vi "Deletar entre Cursores.vi"(8 "error in":errorcluster, 10 "Cluster 3":T1, 11 "WaveformGraph in":refnum<vi>) -> (0 "error out":errorcluster, 2 "output cluster":T1)   [LabVIEW 2020]
uses:
  TypeDef's/Dados consumidor.ctl
  <vilib>/Waveform/WDTOps.llb/WDT Waveform Duration DBL.vi
  <vilib>/Waveform/WDTOps.llb/WDT Get Waveform Subset DBL.vi
  <vilib>/Waveform/WDTOps.llb/WDT Append Waveforms DBL.vi
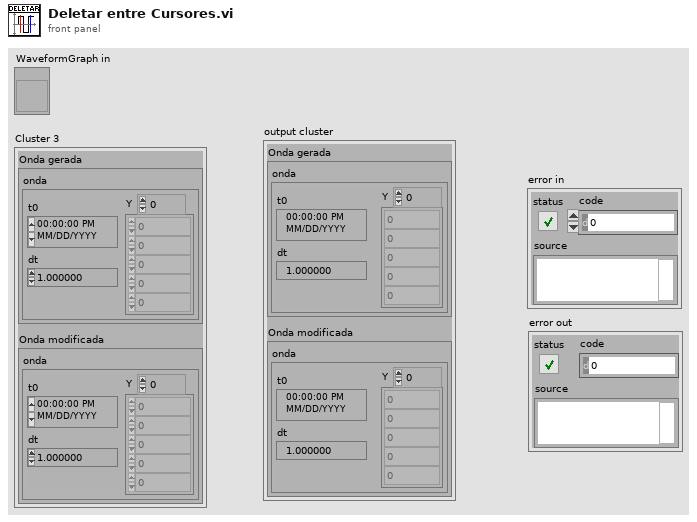
[diagram p1: front panel]
types:
  T1 = typedef "Dados consumidor.ctl" = cluster{"Onda gerada":cluster{"onda":waveform(dbl)}, "Onda modificada":cluster{"onda":waveform(dbl)}}
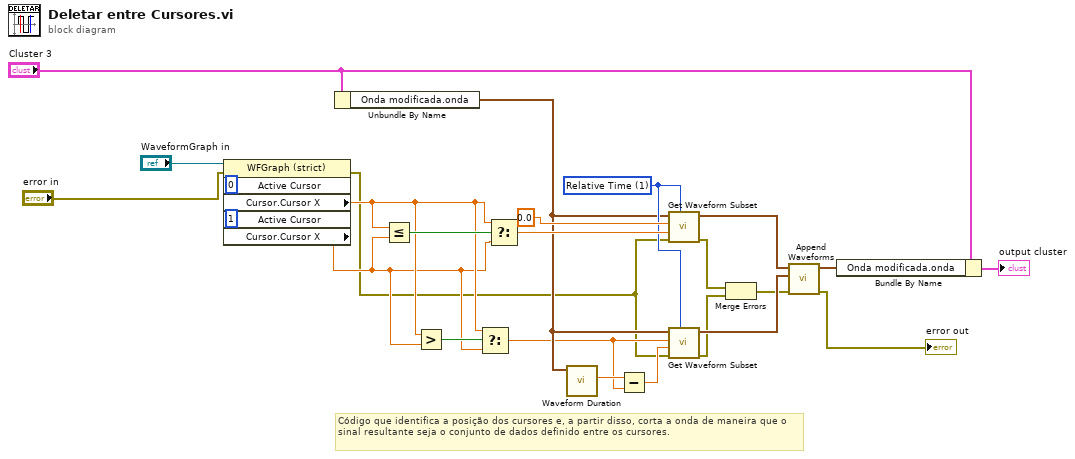
[diagram p0: block diagram]
diagram:
  w15 = u16 1 items=["Samples", "Relative Time"] ("start/duration format")
  # "Código que identifica a posição dos cursores e, a partir disso, corta a onda de maneira que o sinal resultante seja o conjunto de dados definido entre os cursores."
  n1 = property on="Property Node" class="WFGraph (strict)"(reference="WaveformGraph in", error in="error in", "Active Cursor"=u32 0, "Active Cursor"=u32 1) -> (error out=w1:errorcluster, "Cursor.Cursor X"=w13:dbl, "Cursor.Cursor X"=w12:dbl)  [unwired: 1 out]
  n2 = Unbundle By Name("Cluster 3") -> ("Onda modificada.onda"=w9:waveform(dbl))
  n3 = Less Or Equal?(x=w13, y=w12) -> (x <= y?=w20:bool)
  n4 = Greater?(x=w13, y=w12) -> (0:w14:bool)
  n5 = Select(t=w13, s=w14, f=w12) -> (s? t:f=w7:dbl)
  n6 = Select(t=w13, s=w20, f=w12) -> (s? t:f=w24:dbl)
  n7 = call-poly <vilib>:"Waveform Duration.vi"("waveform in"=w9) -> ("duration"=w8:dbl)  [unwired: 8 in, 2 out]
  n8 = Subtract(x=w8, y=w7) -> (x-y=w6:dbl)
  n9 = call-poly <vilib>:"Get Waveform Subset.vi"("start/duration format"=w15, "error in (no error)"=w1, "duration"=w24, "start samples/time"=0.0, "waveform in"=w9) -> ("error out"=w3:errorcluster, "waveform out"=w22:waveform(dbl))  [unwired: 1 in, 2 out]
  n10 = call-poly <vilib>:"Get Waveform Subset.vi"("start/duration format"=w15, "error in (no error)"=w1, "duration"=w6, "start samples/time"=w7, "waveform in"=w9) -> ("error out"=w4:errorcluster, "waveform out"=w11:waveform(dbl))  [unwired: 1 in, 2 out]
  n11 = Merge Errors(w3, w4) -> (w5:errorcluster)
  n12 = call-poly <vilib>:"Append Waveforms.vi"("error in (no error)"=w5, "waveform B"=w11, "waveform A"=w22) -> ("error out"=→"error out":errorcluster, "waveform out"=w10:waveform(dbl))  [unwired: 7 in]
  n13 = Bundle By Name(cluster="Cluster 3", "Onda modificada.onda"=w10) -> (→"output cluster":T1)
